vi "CheckRight.vi"(0 "Chessboard":T2, 5 "ItemIndex":T1, 7 "StoneColor":u16, 11 "error in (no error)":errorcluster) -> (15 "error out":errorcluster)   [LabVIEW 2009]
uses:
  Controls/Chess.ctl
  Controls/ItemIndex.ctl
  RightHaveSameStone.vi
  Controls/directions.ctl
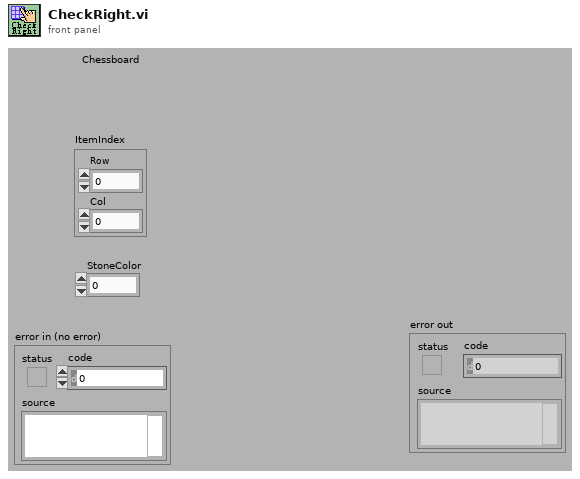
[diagram p1: front panel]
types:
  T1 = typedef "ItemIndex.ctl" = cluster{"Row":i32, "Col":i32}
  T2 = typedef "Chess.ctl" = u16[][]
  T3 = typedef "directions.ctl" = enum16{"Left", "Right", "Top", "Bottom", "TopLeft", "TopRight", "BottomLeft", "BottomRight", "ClearAll", "ReadAll"}
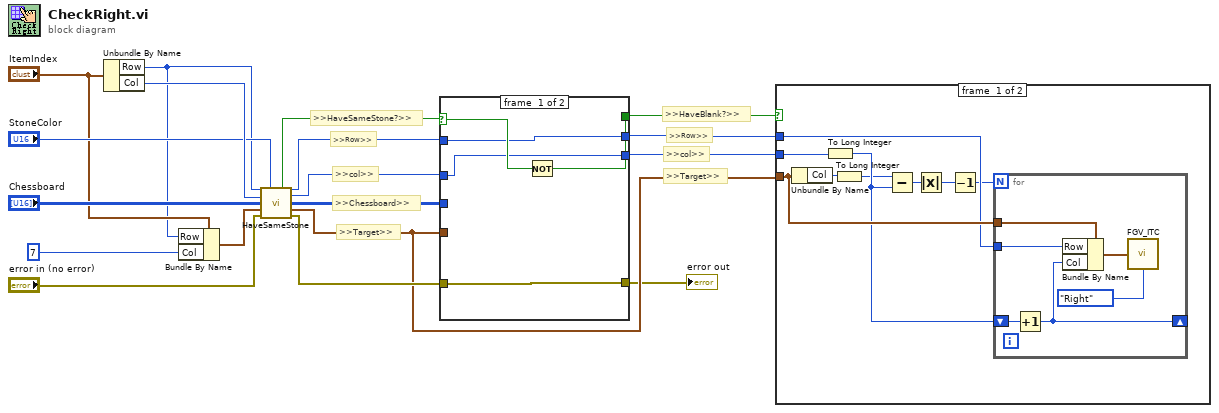
[diagram p0: block diagram]
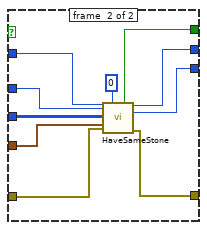
[diagram p3: hidden frame]
diagram:
  # ">>HaveBlank?>>"
  # ">>HaveSameStone?>>"
  # ">>Target>>"
  # ">>col>>"
  # ">>Row>>"
  # ">>Target>>"
  # ">>Chessboard>>"
  # ">>col>>"
  # ">>Row>>"
  n1 = Unbundle By Name("ItemIndex") -> ("Row"=w12:i32, "Col"=w18:i32)
  n2 = Bundle By Name(cluster="ItemIndex", "Row"=w12, "Col"=u32 7) -> (w11:T1)
  n3 = call-poly "HaveSameStone.vi"("Row in"=w12, "StoneColor"="StoneColor", "Col in"=w18, "Chessboard"="Chessboard", "TatgetIndex"=w11, "error in (no error)"="error in (no error)") -> ("HaveSameStone?"=w9:bool, "Row out"=w7:i32, "Col out"=w8:i32, "Chessboard out"=w10:T2, "SSIndex"=w2:T1, "error out"=w6:errorcluster)  [unwired: 4 in]
  n4 = case shown="True" w9 {
    selector: w9 -> [w23 _]
    tunnel: w2 -> [_ w32]
    tunnel: w10 -> [_ w31]
    tunnel: w8 -> [w19 w30]
    tunnel: w7 -> [w20 w29]
    tunnel: w6 -> [w21 w28]
    tunnel: [w22 w27] -> w5
    tunnel: [w21 w26] -> w1
    tunnel: [w20 w25] -> w4
    tunnel: [w19 w24] -> w3
    frame #0 {
      n5 = Not(x=w23) -> (.not. x?=w22:bool)
    }
    frame #1 {
      n6 = call-poly "HaveSameStone.vi"("Row in"=w29, "StoneColor"=u16 0, "Col in"=w30, "Chessboard"=w31, "TatgetIndex"=w32, "error in (no error)"=w28) -> ("HaveSameStone?"=w27:bool, "Row out"=w25:i32, "Col out"=w24:i32, "error out"=w26:errorcluster)  [unwired: 4 in, 2 out]
    }
  }
  "error out" <- w1
  n7 = case shown="False" w5 {
    tunnel: w4 -> [w41 _]
    tunnel: w3 -> [w40 _]
    tunnel: w2 -> [w42 _]
    frame #0 {
      n8 = Unbundle By Name(w42) -> ("Col"=w38:i32)
      n9 = To Long Integer(number=w40) -> (32bit integer=w39:i32)
      n10 = To Long Integer(number=w38) -> (32bit integer=w37:i32)
      n11 = Subtract(x=w37, y=w39) -> (x-y=w36:i32)
      n12 = Absolute Value(x=w36) -> (abs(x)=w35:i32)
      n13 = Decrement(x=w35) -> (x-1=w34:i32)
      n14 = for {
        N: w34 -> [_]
        shift-right: [w45] -> _
        shift-left: w39 -> [w48]
        tunnel: w42 -> [w47]
        tunnel: w41 -> [w46]
        n15 = Increment(x=w48) -> (x+1=w45:i32)
        n16 = Bundle By Name(cluster=w47, "Row"=w46, "Col"=w45) -> (w44:T1)
        n17 = call "FGV_ITC.vi"("ItemIndex"=w44, "Action"=directions."Right") -> ()  [unwired: 12 in, 2 out]
      }
    }
    frame #1 {
    }
  }
